vi "Prepare Config Data for Save.vi"(8 "error in (no error)":errorcluster, 10 "Shutdown Data":T3, 11 "Settings in":refnum<class "Settings.lvclass">) -> (0 "error out":errorcluster, 2 "Config Data":T1={"DS First Launch"=FALSE, "LogBaseFolder"=path "", "Live Logging"=FALSE, "Server Port"=0, "Max Number ML Rows"=0, "AM.WinBounds"={"Left"=0, "Top"=0, "Right"=0, "Bottom"=0}, "AM.FP.State"=enum."Invalid", "AM.Monitor"=0, "AM.Column Widths"=[], "ML.Visible Columns"=[], "ML.Splitter Position"=0, "ML.Column Widths"=[], "ML.WinBounds"={"Left"=0, "Top"=0, "Right"=0, "Bottom"=0}, "ML.FP.State"=enum."Invalid", "ML.Monitor"=0}, 3 "Settings out":refnum<class "Settings.lvclass">)   [LabVIEW 2017, in "Settings.lvclass"]
uses:
  Settings.lvclass
  rqp_Receive Shutdown Data.ctl
  <vilib>/Utility/miscctls.llb/LVRectTypeDef.ctl
  Config Data.ctl
  Settings.lvclass/Settings.ctl
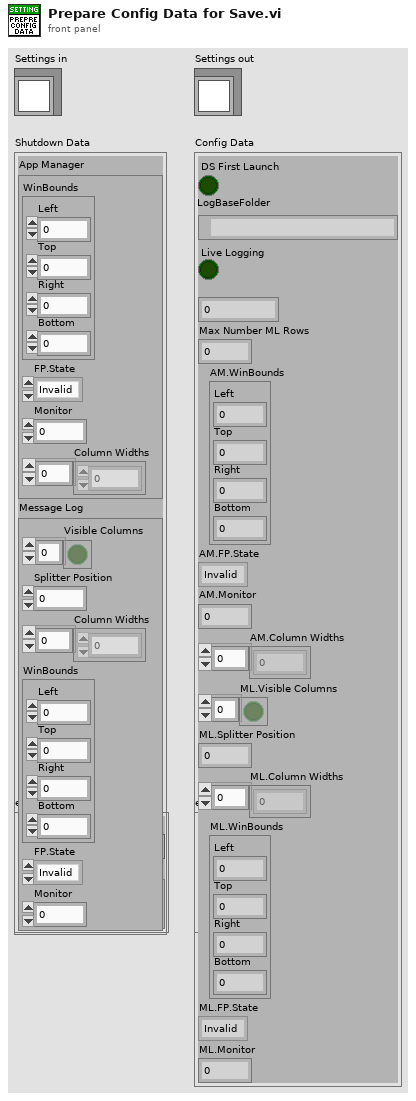
[diagram p1: front panel]
types:
  T1 = typedef "Settings.lvclass/Config Data.ctl" = cluster{"DS First Launch":bool, "LogBaseFolder":path, "Live Logging":bool, "Server Port":u16, "Max Number ML Rows":i32, "AM.WinBounds":T2, "AM.FP.State":enum32{"Invalid", "Standard", "Closed", "Hidden", "Minimized", "Maximized"}, "AM.Monitor":u16, "AM.Column Widths":u32[], "ML.Visible Columns":bool[], "ML.Splitter Position":i32, "ML.Column Widths":u32[], "ML.WinBounds":T2, "ML.FP.State":enum32{"Invalid", "Standard", "Closed", "Hidden", "Minimized", "Maximized"}, "ML.Monitor":u16}
  T2 = typedef "LVRectTypeDef.ctl" = cluster{"Left":i16, "Top":i16, "Right":i16, "Bottom":i16}
  T3 = typedef "Settings.lvclass/rqp_Receive Shutdown Data.ctl" = cluster{"App Manager":cluster{"WinBounds":T2, "FP.State":enum32{"Invalid", "Standard", "Closed", "Hidden", "Minimized", "Maximized"}, "Monitor":u16, "Column Widths":u32[]}, "Message Log":cluster{"Visible Columns":bool[], "Splitter Position":i32, "Column Widths":u32[], "WinBounds":T2, "FP.State":enum32{"Invalid", "Standard", "Closed", "Hidden", "Minimized", "Maximized"}, "Monitor":u16}}
  T4 = cluster{"Visible Columns":bool[], "Splitter Position":i32, "Column Widths":u32[], "WinBounds":T2, "FP.State":enum32{"Invalid", "Standard", "Closed", "Hidden", "Minimized", "Maximized"}, "Monitor":u16}
  T5 = cluster{"WinBounds":T2, "FP.State":enum32{"Invalid", "Standard", "Closed", "Hidden", "Minimized", "Maximized"}, "Monitor":u16, "Column Widths":u32[]}
  T6 = enum32{"Invalid", "Standard", "Closed", "Hidden", "Minimized", "Maximized"}
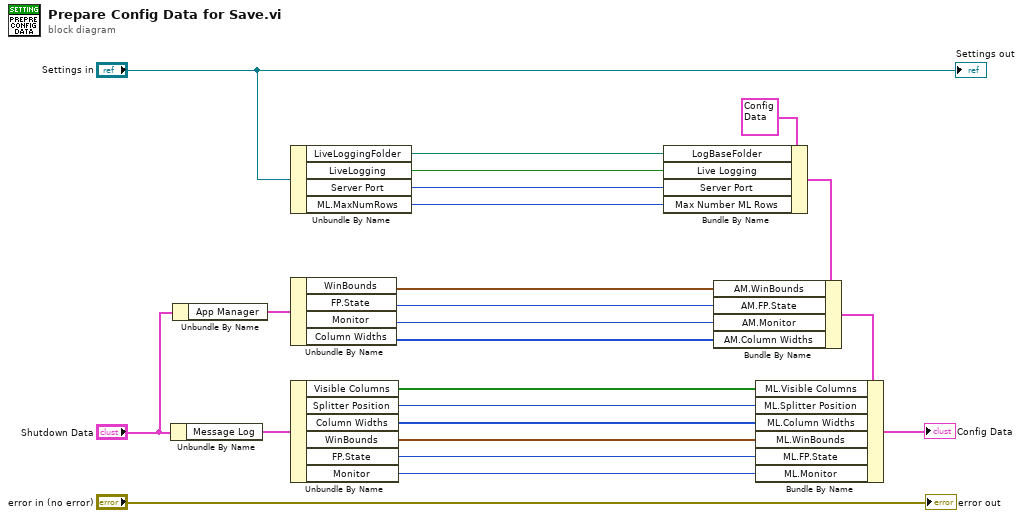
[diagram p0: block diagram]
diagram:
  n1 = Unbundle By Name("Shutdown Data") -> ("Message Log"=w22:T4)
  n2 = Unbundle By Name("Shutdown Data") -> ("App Manager"=w23:T5)
  n3 = Unbundle By Name("Settings in") -> ("LiveLoggingFolder"=w18:path, "LiveLogging"=w17:bool, "Server Port"=w19:u16, "ML.MaxNumRows"=w9:u16)
  n4 = Unbundle By Name(w23) -> ("WinBounds"=w15:T2, "FP.State"=w14:T6, "Monitor"=w13:u16, "Column Widths"=w12:u32[])
  n5 = Unbundle By Name(w22) -> ("Visible Columns"=w8:bool[], "Splitter Position"=w7:i32, "Column Widths"=w6:u32[], "WinBounds"=w4:T2, "FP.State"=w3:T6, "Monitor"=w2:u16)
  n6 = Bundle By Name(cluster=T1 {"DS First Launch"=FALSE, "LogBaseFolder"=path "", "Live Logging"=FALSE, "Server Port"=0, "Max Number ML Rows"=0, "AM.WinBounds"={"Left"=0, "Top"=0, "Right"=0, "Bottom"=0}, "AM.FP.State"=enum."Invalid", "AM.Monitor"=0, "AM.Column Widths"=[], "ML.Visible Columns"=[], "ML.Splitter Position"=0, "ML.Column Widths"=[], "ML.WinBounds"={"Left"=0, "Top"=0, "Right"=0, "Bottom"=0}, "ML.FP.State"=enum."Invalid", "ML.Monitor"=0} ("Config Data"), "LogBaseFolder"=w18, "Live Logging"=w17, "Server Port"=w19, "Max Number ML Rows"=w9) -> (w16:T1)
  n7 = Bundle By Name(cluster=w16, "AM.WinBounds"=w15, "AM.FP.State"=w14, "AM.Monitor"=w13, "AM.Column Widths"=w12) -> (w11:T1)
  n8 = Bundle By Name(cluster=w11, "ML.Visible Columns"=w8, "ML.Splitter Position"=w7, "ML.Column Widths"=w6, "ML.WinBounds"=w4, "ML.FP.State"=w3, "ML.Monitor"=w2) -> (→"Config Data":T1)
  "error out" <- "error in (no error)"
  "Settings out" <- "Settings in"
